vi "PXI Power Control.vi"(1 "Enable Relays":bool, 2 "Reset IO":bool, 3 "error in (no error)":errorcluster {"code" format="%.0x"}, 4 "Enum":T2(ring), 5 "topology name":T1="2566/16-SPDT", 6 "resource name":refnum<k15>="PXI1Slot6") -> (0 "error out":errorcluster)   [LabVIEW 2014]
uses:
  <instrlib>/niSwitch/niswitch.llb/niSwitch Relay Action.ctl
  <instrlib>/niSwitch/niswitch.llb/niSwitch Topologies.ctl
panel:
  out "instrument handle out":refnum<k15>
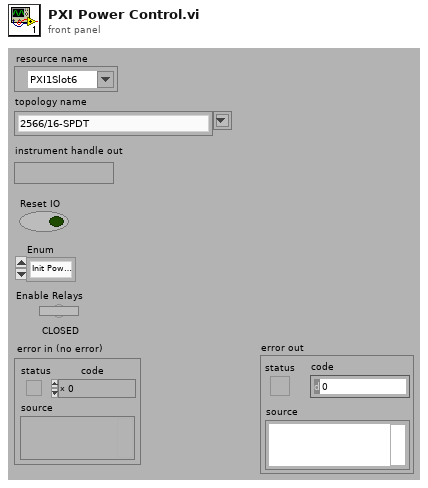
[diagram p1: front panel]
types:
  T1 = typedef "niSwitch Topologies.ctl" = string
  T2 = enum16{"Init Power Relays", "Primary Sense", "Battery Sense", "Primary Power", "Battery Power", "Secondary Power", "Auxillary Power", "DeInit Power Relays"}
  T3 = typedef "niSwitch Relay Action.ctl" = i32
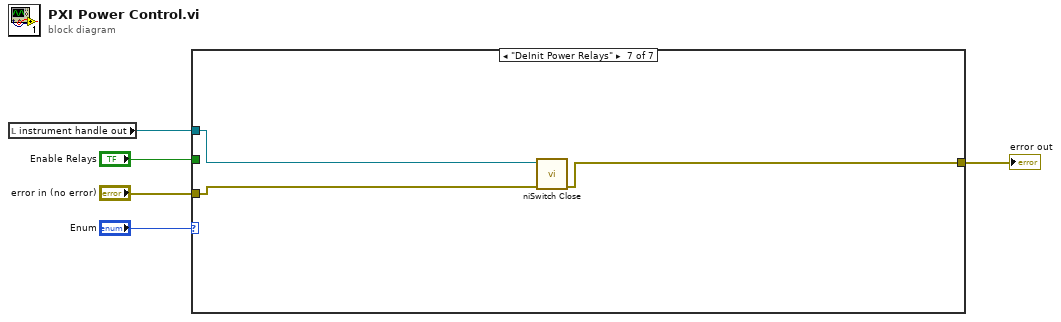
[diagram p0: block diagram]
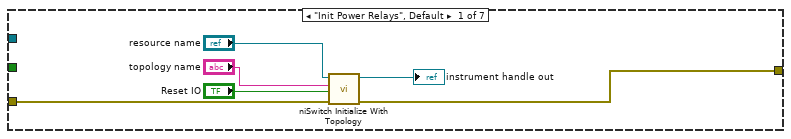
[diagram p2: hidden frame]
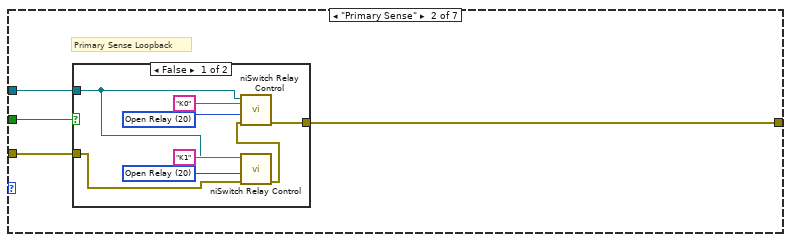
[diagram p3: hidden frame]
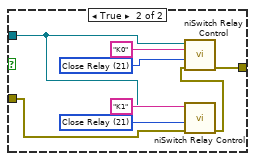
[diagram p4: hidden frame]
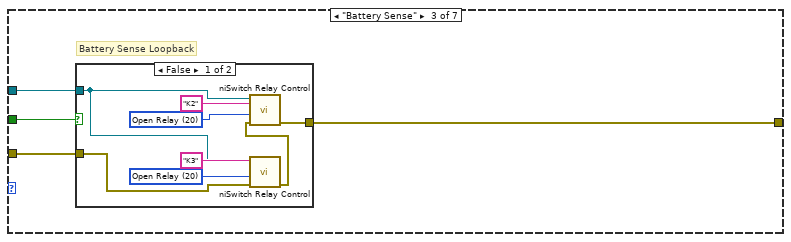
[diagram p5: hidden frame]
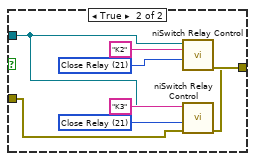
[diagram p6: hidden frame]
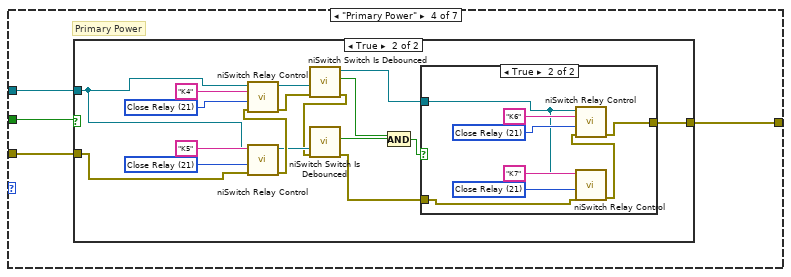
[diagram p7: hidden frame]
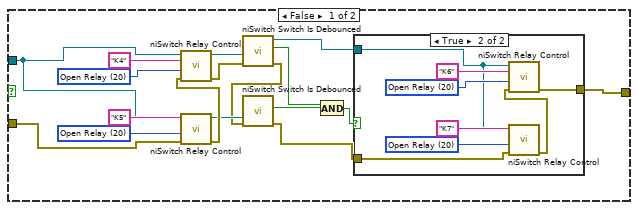
[diagram p8: hidden frame]
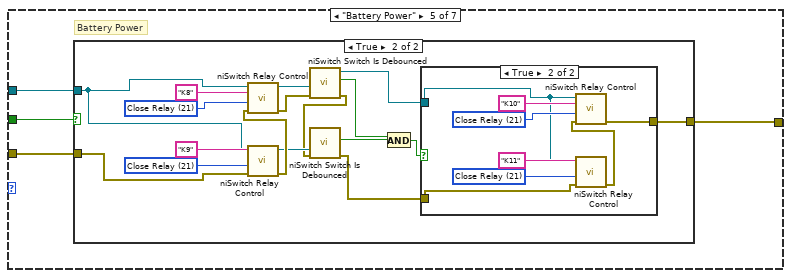
[diagram p11: hidden frame]
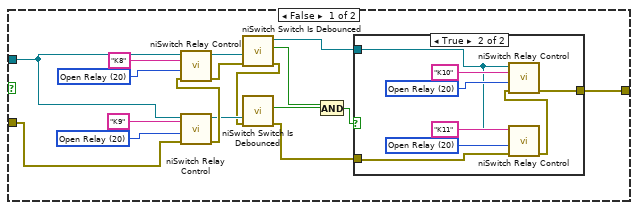
[diagram p12: hidden frame]
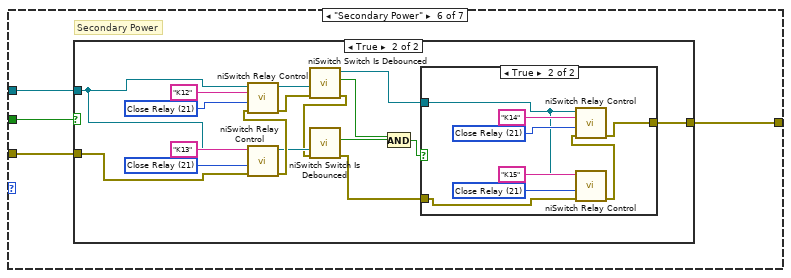
[diagram p15: hidden frame]
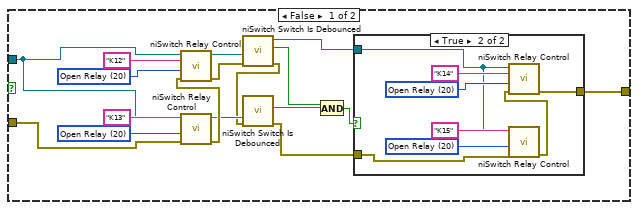
[diagram p16: hidden frame]
diagram:
  n1 = local read "instrument handle out"() -> (w4:refnum<k15>)
  n2 = case shown="\"DeInit Power Relays\"" "Enum" {
    tunnel: w4 -> [_ w15 w35 w55 w111 w167 w222]
    tunnel: [w11 w14 w32 w53 w110 w164 w220] -> w3
    tunnel: "Enable Relays" -> [_ w13 w34 w54 w109 w166 _]
    tunnel: "error in (no error)" -> [w10 w12 w33 w52 w108 w165 w221]
    frame "Init Power Relays", Default {
      n3 = call <instrlib>:"niSwitch Initialize With Topology.vi"("error in (no error)"=w10, "reset device (boolean value)"="Reset IO", "topology name"="topology name", "resource name"="resource name") -> ("error out"=w11:errorcluster, "instrument handle out"=→"instrument handle out":refnum<k15>)  [unwired: 6 in]
    }
    frame "Primary Sense" {
      # "Primary Sense Loopback"
      n4 = case shown="False" w13 {
        tunnel: [w21 w29] -> w14
        tunnel: w15 -> [w16 w24]
        tunnel: w12 -> [w17 w25]
        frame False {
          w20 = T3 20 items=["Open Relay"=20, "Close Relay"=21] ("relay action (Close Relay)")
          w23 = T3 20 items=["Open Relay"=20, "Close Relay"=21] ("relay action (Close Relay)")
          n5 = call <instrlib>:"niSwitch Relay Control.vi"("error in (no error)"=w17, "relay action (Close Relay)"=w20, "relay name"="K1", "instrument handle"=w16) -> ("error out"=w18:errorcluster)  [unwired: 6 in, 1 out]
          n6 = call <instrlib>:"niSwitch Relay Control.vi"("error in (no error)"=w18, "relay action (Close Relay)"=w23, "relay name"="K0", "instrument handle"=w16) -> ("error out"=w21:errorcluster)  [unwired: 6 in, 1 out]
        }
        frame True {
          w28 = T3 21 items=["Open Relay"=20, "Close Relay"=21] ("relay action (Close Relay)")
          w31 = T3 21 items=["Open Relay"=20, "Close Relay"=21] ("relay action (Close Relay)")
          n7 = call <instrlib>:"niSwitch Relay Control.vi"("error in (no error)"=w25, "relay action (Close Relay)"=w28, "relay name"="K1", "instrument handle"=w24) -> ("error out"=w26:errorcluster)  [unwired: 6 in, 1 out]
          n8 = call <instrlib>:"niSwitch Relay Control.vi"("error in (no error)"=w26, "relay action (Close Relay)"=w31, "relay name"="K0", "instrument handle"=w24) -> ("error out"=w29:errorcluster)  [unwired: 6 in, 1 out]
        }
      }
    }
    frame "Battery Sense" {
      # "Battery Sense Loopback"
      n9 = case shown="False" w34 {
        tunnel: w35 -> [w38 w46]
        tunnel: [w41 w49] -> w32
        tunnel: w33 -> [w36 w44]
        frame False {
          w40 = T3 20 items=["Open Relay"=20, "Close Relay"=21] ("relay action (Close Relay)")
          w43 = T3 20 items=["Open Relay"=20, "Close Relay"=21] ("relay action (Close Relay)")
          n10 = call <instrlib>:"niSwitch Relay Control.vi"("error in (no error)"=w36, "relay action (Close Relay)"=w40, "relay name"="K3", "instrument handle"=w38) -> ("error out"=w37:errorcluster)  [unwired: 6 in, 1 out]
          n11 = call <instrlib>:"niSwitch Relay Control.vi"("error in (no error)"=w37, "relay action (Close Relay)"=w43, "relay name"="K2", "instrument handle"=w38) -> ("error out"=w41:errorcluster)  [unwired: 6 in, 1 out]
        }
        frame True {
          w48 = T3 21 items=["Open Relay"=20, "Close Relay"=21] ("relay action (Close Relay)")
          w51 = T3 21 items=["Open Relay"=20, "Close Relay"=21] ("relay action (Close Relay)")
          n12 = call <instrlib>:"niSwitch Relay Control.vi"("error in (no error)"=w44, "relay action (Close Relay)"=w48, "relay name"="K3", "instrument handle"=w46) -> ("error out"=w45:errorcluster)  [unwired: 6 in, 1 out]
          n13 = call <instrlib>:"niSwitch Relay Control.vi"("error in (no error)"=w45, "relay action (Close Relay)"=w51, "relay name"="K2", "instrument handle"=w46) -> ("error out"=w49:errorcluster)  [unwired: 6 in, 1 out]
        }
      }
    }
    frame "Primary Power" {
      # "Primary Power"
      n14 = case shown="True" w54 {
        tunnel: w55 -> [w61 w94]
        tunnel: [w57 w83] -> w53
        tunnel: w52 -> [w56 w82]
        frame False {
          w70 = T3 20 items=["Open Relay"=20, "Close Relay"=21] ("relay action (Close Relay)")
          w72 = T3 20 items=["Open Relay"=20, "Close Relay"=21] ("relay action (Close Relay)")
          n15 = call <instrlib>:"niSwitch Relay Control.vi"("error in (no error)"=w56, "relay action (Close Relay)"=w70, "relay name"="K5", "instrument handle"=w61) -> ("error out"=w68:errorcluster, "instrument handle out"=w66:refnum<k15>)  [unwired: 6 in]
          n16 = call <instrlib>:"niSwitch Relay Control.vi"("error in (no error)"=w68, "relay action (Close Relay)"=w72, "relay name"="K4", "instrument handle"=w61) -> ("error out"=w60:errorcluster, "instrument handle out"=w67:refnum<k15>)  [unwired: 6 in]
          n17 = call <instrlib>:"niSwitch Switch Is Debounced.vi"("error in (no error)"=w60, "instrument handle"=w67) -> ("error out"=w59:errorcluster, "is debounced"=w64:bool, "instrument handle out"=w62:refnum<k15>)  [unwired: 7 in]
          n18 = call <instrlib>:"niSwitch Switch Is Debounced.vi"("error in (no error)"=w59, "instrument handle"=w66) -> ("error out"=w58:errorcluster, "is debounced"=w65:bool)  [unwired: 7 in, 1 out]
          n19 = And(x=w64, y=w65) -> (x .and. y?=w63:bool)
          n20 = case shown="True" w63 {
            tunnel: w62 -> [_ w76]
            tunnel: w58 -> [w73 w75]
            tunnel: [w73 w74] -> w57
            frame False {
            }
            frame True {
              w79 = T3 20 items=["Open Relay"=20, "Close Relay"=21] ("relay action (Close Relay)")
              w81 = T3 20 items=["Open Relay"=20, "Close Relay"=21] ("relay action (Close Relay)")
              n21 = call <instrlib>:"niSwitch Relay Control.vi"("error in (no error)"=w75, "relay action (Close Relay)"=w79, "relay name"="K7", "instrument handle"=w76) -> ("error out"=w77:errorcluster)  [unwired: 6 in, 1 out]
              n22 = call <instrlib>:"niSwitch Relay Control.vi"("error in (no error)"=w77, "relay action (Close Relay)"=w81, "relay name"="K6", "instrument handle"=w76) -> ("error out"=w74:errorcluster)  [unwired: 6 in, 1 out]
            }
          }
        }
        frame True {
          w96 = T3 21 items=["Open Relay"=20, "Close Relay"=21] ("relay action (Close Relay)")
          w98 = T3 21 items=["Open Relay"=20, "Close Relay"=21] ("relay action (Close Relay)")
          n23 = call <instrlib>:"niSwitch Relay Control.vi"("error in (no error)"=w82, "relay action (Close Relay)"=w96, "relay name"="K5", "instrument handle"=w94) -> ("error out"=w93:errorcluster, "instrument handle out"=w91:refnum<k15>)  [unwired: 6 in]
          n24 = call <instrlib>:"niSwitch Relay Control.vi"("error in (no error)"=w93, "relay action (Close Relay)"=w98, "relay name"="K4", "instrument handle"=w94) -> ("error out"=w86:errorcluster, "instrument handle out"=w92:refnum<k15>)  [unwired: 6 in]
          n25 = call <instrlib>:"niSwitch Switch Is Debounced.vi"("error in (no error)"=w86, "instrument handle"=w92) -> ("error out"=w85:errorcluster, "is debounced"=w89:bool, "instrument handle out"=w87:refnum<k15>)  [unwired: 7 in]
          n26 = call <instrlib>:"niSwitch Switch Is Debounced.vi"("error in (no error)"=w85, "instrument handle"=w91) -> ("error out"=w84:errorcluster, "is debounced"=w90:bool)  [unwired: 7 in, 1 out]
          n27 = And(x=w89, y=w90) -> (x .and. y?=w88:bool)
          n28 = case shown="True" w88 {
            tunnel: w87 -> [_ w102]
            tunnel: w84 -> [w99 w101]
            tunnel: [w99 w100] -> w83
            frame False {
            }
            frame True {
              w105 = T3 21 items=["Open Relay"=20, "Close Relay"=21] ("relay action (Close Relay)")
              w107 = T3 21 items=["Open Relay"=20, "Close Relay"=21] ("relay action (Close Relay)")
              n29 = call <instrlib>:"niSwitch Relay Control.vi"("error in (no error)"=w101, "relay action (Close Relay)"=w105, "relay name"="K7", "instrument handle"=w102) -> ("error out"=w103:errorcluster)  [unwired: 6 in, 1 out]
              n30 = call <instrlib>:"niSwitch Relay Control.vi"("error in (no error)"=w103, "relay action (Close Relay)"=w107, "relay name"="K6", "instrument handle"=w102) -> ("error out"=w100:errorcluster)  [unwired: 6 in, 1 out]
            }
          }
        }
      }
    }
    frame "Battery Power" {
      # "Battery Power"
      n31 = case shown="True" w109 {
        tunnel: w111 -> [w117 w143]
        tunnel: [w113 w142] -> w110
        tunnel: w108 -> [w112 w138]
        frame False {
          w126 = T3 20 items=["Open Relay"=20, "Close Relay"=21] ("relay action (Close Relay)")
          w128 = T3 20 items=["Open Relay"=20, "Close Relay"=21] ("relay action (Close Relay)")
          n32 = call <instrlib>:"niSwitch Relay Control.vi"("error in (no error)"=w112, "relay action (Close Relay)"=w126, "relay name"="K9", "instrument handle"=w117) -> ("error out"=w124:errorcluster, "instrument handle out"=w122:refnum<k15>)  [unwired: 6 in]
          n33 = call <instrlib>:"niSwitch Relay Control.vi"("error in (no error)"=w124, "relay action (Close Relay)"=w128, "relay name"="K8", "instrument handle"=w117) -> ("error out"=w116:errorcluster, "instrument handle out"=w123:refnum<k15>)  [unwired: 6 in]
          n34 = call <instrlib>:"niSwitch Switch Is Debounced.vi"("error in (no error)"=w116, "instrument handle"=w123) -> ("error out"=w115:errorcluster, "is debounced"=w120:bool, "instrument handle out"=w118:refnum<k15>)  [unwired: 7 in]
          n35 = call <instrlib>:"niSwitch Switch Is Debounced.vi"("error in (no error)"=w115, "instrument handle"=w122) -> ("error out"=w114:errorcluster, "is debounced"=w121:bool)  [unwired: 7 in, 1 out]
          n36 = And(x=w120, y=w121) -> (x .and. y?=w119:bool)
          n37 = case shown="True" w119 {
            tunnel: w118 -> [_ w132]
            tunnel: w114 -> [w129 w131]
            tunnel: [w129 w130] -> w113
            frame False {
            }
            frame True {
              w135 = T3 20 items=["Open Relay"=20, "Close Relay"=21] ("relay action (Close Relay)")
              w137 = T3 20 items=["Open Relay"=20, "Close Relay"=21] ("relay action (Close Relay)")
              n38 = call <instrlib>:"niSwitch Relay Control.vi"("error in (no error)"=w131, "relay action (Close Relay)"=w135, "relay name"="K11", "instrument handle"=w132) -> ("error out"=w133:errorcluster)  [unwired: 6 in, 1 out]
              n39 = call <instrlib>:"niSwitch Relay Control.vi"("error in (no error)"=w133, "relay action (Close Relay)"=w137, "relay name"="K10", "instrument handle"=w132) -> ("error out"=w130:errorcluster)  [unwired: 6 in, 1 out]
            }
          }
        }
        frame True {
          w152 = T3 21 items=["Open Relay"=20, "Close Relay"=21] ("relay action (Close Relay)")
          w154 = T3 21 items=["Open Relay"=20, "Close Relay"=21] ("relay action (Close Relay)")
          n40 = call <instrlib>:"niSwitch Relay Control.vi"("error in (no error)"=w138, "relay action (Close Relay)"=w152, "relay name"="K9", "instrument handle"=w143) -> ("error out"=w150:errorcluster, "instrument handle out"=w148:refnum<k15>)  [unwired: 6 in]
          n41 = call <instrlib>:"niSwitch Relay Control.vi"("error in (no error)"=w150, "relay action (Close Relay)"=w154, "relay name"="K8", "instrument handle"=w143) -> ("error out"=w141:errorcluster, "instrument handle out"=w149:refnum<k15>)  [unwired: 6 in]
          n42 = call <instrlib>:"niSwitch Switch Is Debounced.vi"("error in (no error)"=w141, "instrument handle"=w149) -> ("error out"=w140:errorcluster, "is debounced"=w146:bool, "instrument handle out"=w144:refnum<k15>)  [unwired: 7 in]
          n43 = call <instrlib>:"niSwitch Switch Is Debounced.vi"("error in (no error)"=w140, "instrument handle"=w148) -> ("error out"=w139:errorcluster, "is debounced"=w147:bool)  [unwired: 7 in, 1 out]
          n44 = And(x=w146, y=w147) -> (x .and. y?=w145:bool)
          n45 = case shown="True" w145 {
            tunnel: w144 -> [_ w158]
            tunnel: [w155 w157] -> w142
            tunnel: w139 -> [w155 w156]
            frame False {
            }
            frame True {
              w161 = T3 21 items=["Open Relay"=20, "Close Relay"=21] ("relay action (Close Relay)")
              w163 = T3 21 items=["Open Relay"=20, "Close Relay"=21] ("relay action (Close Relay)")
              n46 = call <instrlib>:"niSwitch Relay Control.vi"("error in (no error)"=w156, "relay action (Close Relay)"=w161, "relay name"="K11", "instrument handle"=w158) -> ("error out"=w159:errorcluster)  [unwired: 6 in, 1 out]
              n47 = call <instrlib>:"niSwitch Relay Control.vi"("error in (no error)"=w159, "relay action (Close Relay)"=w163, "relay name"="K10", "instrument handle"=w158) -> ("error out"=w157:errorcluster)  [unwired: 6 in, 1 out]
            }
          }
        }
      }
    }
    frame "Secondary Power" {
      # "Secondary Power"
      n48 = case shown="True" w166 {
        tunnel: w167 -> [w173 w195]
        tunnel: w165 -> [w172 w194]
        tunnel: [w171 w196] -> w164
        frame False {
          w182 = T3 20 items=["Open Relay"=20, "Close Relay"=21] ("relay action (Close Relay)")
          w184 = T3 20 items=["Open Relay"=20, "Close Relay"=21] ("relay action (Close Relay)")
          n49 = call <instrlib>:"niSwitch Relay Control.vi"("error in (no error)"=w172, "relay action (Close Relay)"=w182, "relay name"="K13", "instrument handle"=w173) -> ("error out"=w180:errorcluster, "instrument handle out"=w178:refnum<k15>)  [unwired: 6 in]
          n50 = call <instrlib>:"niSwitch Relay Control.vi"("error in (no error)"=w180, "relay action (Close Relay)"=w184, "relay name"="K12", "instrument handle"=w173) -> ("error out"=w170:errorcluster, "instrument handle out"=w179:refnum<k15>)  [unwired: 6 in]
          n51 = call <instrlib>:"niSwitch Switch Is Debounced.vi"("error in (no error)"=w170, "instrument handle"=w179) -> ("error out"=w169:errorcluster, "is debounced"=w176:bool, "instrument handle out"=w174:refnum<k15>)  [unwired: 7 in]
          n52 = call <instrlib>:"niSwitch Switch Is Debounced.vi"("error in (no error)"=w169, "instrument handle"=w178) -> ("error out"=w168:errorcluster, "is debounced"=w177:bool)  [unwired: 7 in, 1 out]
          n53 = And(x=w176, y=w177) -> (x .and. y?=w175:bool)
          n54 = case shown="True" w175 {
            tunnel: w174 -> [_ w188]
            tunnel: [w185 w187] -> w171
            tunnel: w168 -> [w185 w186]
            frame False {
            }
            frame True {
              w191 = T3 20 items=["Open Relay"=20, "Close Relay"=21] ("relay action (Close Relay)")
              w193 = T3 20 items=["Open Relay"=20, "Close Relay"=21] ("relay action (Close Relay)")
              n55 = call <instrlib>:"niSwitch Relay Control.vi"("error in (no error)"=w186, "relay action (Close Relay)"=w191, "relay name"="K15", "instrument handle"=w188) -> ("error out"=w189:errorcluster)  [unwired: 6 in, 1 out]
              n56 = call <instrlib>:"niSwitch Relay Control.vi"("error in (no error)"=w189, "relay action (Close Relay)"=w193, "relay name"="K14", "instrument handle"=w188) -> ("error out"=w187:errorcluster)  [unwired: 6 in, 1 out]
            }
          }
        }
        frame True {
          w208 = T3 21 items=["Open Relay"=20, "Close Relay"=21] ("relay action (Close Relay)")
          w210 = T3 21 items=["Open Relay"=20, "Close Relay"=21] ("relay action (Close Relay)")
          n57 = call <instrlib>:"niSwitch Relay Control.vi"("error in (no error)"=w194, "relay action (Close Relay)"=w208, "relay name"="K13", "instrument handle"=w195) -> ("error out"=w206:errorcluster, "instrument handle out"=w204:refnum<k15>)  [unwired: 6 in]
          n58 = call <instrlib>:"niSwitch Relay Control.vi"("error in (no error)"=w206, "relay action (Close Relay)"=w210, "relay name"="K12", "instrument handle"=w195) -> ("error out"=w199:errorcluster, "instrument handle out"=w205:refnum<k15>)  [unwired: 6 in]
          n59 = call <instrlib>:"niSwitch Switch Is Debounced.vi"("error in (no error)"=w199, "instrument handle"=w205) -> ("error out"=w198:errorcluster, "is debounced"=w202:bool, "instrument handle out"=w200:refnum<k15>)  [unwired: 7 in]
          n60 = call <instrlib>:"niSwitch Switch Is Debounced.vi"("error in (no error)"=w198, "instrument handle"=w204) -> ("error out"=w197:errorcluster, "is debounced"=w203:bool)  [unwired: 7 in, 1 out]
          n61 = And(x=w202, y=w203) -> (x .and. y?=w201:bool)
          n62 = case shown="True" w201 {
            tunnel: w200 -> [_ w214]
            tunnel: w197 -> [w211 w213]
            tunnel: [w211 w212] -> w196
            frame False {
            }
            frame True {
              w217 = T3 21 items=["Open Relay"=20, "Close Relay"=21] ("relay action (Close Relay)")
              w219 = T3 21 items=["Open Relay"=20, "Close Relay"=21] ("relay action (Close Relay)")
              n63 = call <instrlib>:"niSwitch Relay Control.vi"("error in (no error)"=w213, "relay action (Close Relay)"=w217, "relay name"="K15", "instrument handle"=w214) -> ("error out"=w215:errorcluster)  [unwired: 6 in, 1 out]
              n64 = call <instrlib>:"niSwitch Relay Control.vi"("error in (no error)"=w215, "relay action (Close Relay)"=w219, "relay name"="K14", "instrument handle"=w214) -> ("error out"=w212:errorcluster)  [unwired: 6 in, 1 out]
            }
          }
        }
      }
    }
    frame "DeInit Power Relays" {
      n65 = call <instrlib>:"niSwitch Close.vi"("error in (no error)"=w221, "instrument handle"=w222) -> ("error out"=w220:errorcluster)  [unwired: 9 in]
    }
  }
  "error out" <- w3
